vi "dfd_MRate_Calculate CIC MSB Pos and Gain.vi"(5 "#stage":i32, 6 "Decimation? (T)":bool, 7 "lag":i32, 11 "factor":i32) -> (1 "filter gain":dbl, 3 "bit growth":i16)   [LabVIEW 2017, in "NI_DigFilter_FXP.lvlib"]
uses:
  <vilib>/addons/Digital Filter Design/NI_DigFilter_FXP.lvlib
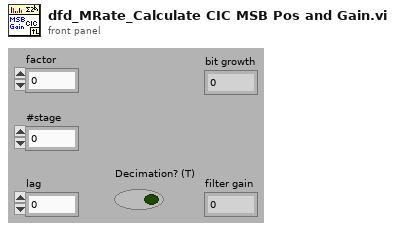
[diagram p1: front panel]
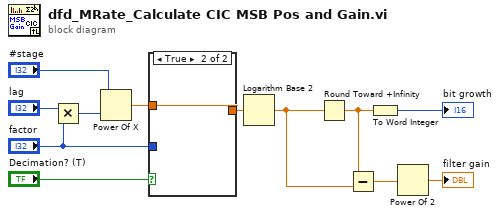
[diagram p0: block diagram]
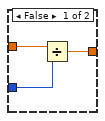
[diagram p2: hidden frame]
diagram:
  n1 = Multiply(x="lag", y="factor") -> (x*y=w7:i32)
  n2 = Power Of X(1:w7, 2:"#stage") -> (0:w5:dbl)
  n3 = case shown="True" "Decimation? (T)" {
    tunnel: w5 -> [w15 w16]
    tunnel: "factor" -> [w14 _]
    tunnel: [w13 w16] -> w2
    frame False {
      n4 = Divide(x=w15, y=w14) -> (x/y=w13:dbl)
    }
    frame True {
    }
  }
  n5 = Logarithm Base 2(1:w2) -> (0:w1:dbl)
  n6 = Round Toward +Infinity(x=w1) -> (ceil(x): smallest int >= x=w9:dbl)
  n7 = Subtract(x=w9, y=w1) -> (x-y=w10:dbl)
  n8 = To Word Integer(number=w9) -> (16bit integer=→"bit growth":i16)
  n9 = Power Of 2(x=w10) -> (2^x=→"filter gain":dbl)
